vi "MagX Get Info From Server.vi"(6 "Save cache":bool, 7 "url":string="http://magx.lanl.gov/rest/now/", 8 "error in":errorcluster, 9 "Use cache":bool, 10 "Local cache  file":path=path "C:/Data/tmp/calendar.json", 11 "Station":string="Cell_3") -> (0 "error out":errorcluster, 2 "Online":bool, 3 "body":string)   [LabVIEW 2024]
uses:
  <vilib>/Utility/error.llb/Error Cluster From Error Code.vi
  <vilib>/ErrorRing/Error Ring.xnode
  <vilib>/httpClient/LabVIEWHTTPClient.lvlib
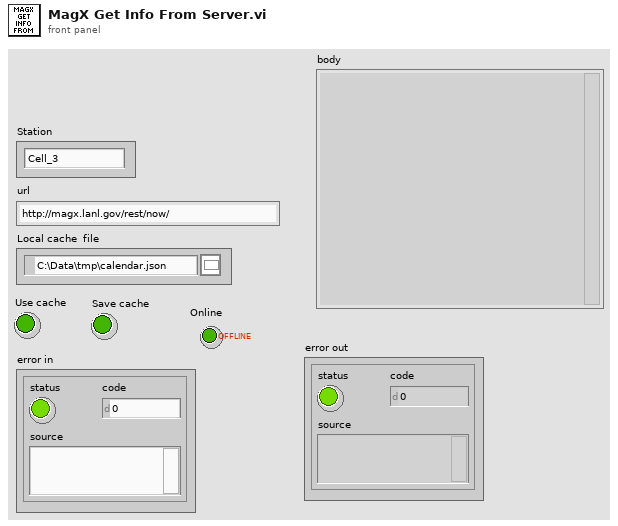
[diagram p1: front panel]
types:
  T1 = typedef "LabVIEWHTTPClient.lvlib/ClientHandle.ctl" = refnum<k1>
  T2 = enum16{"open", "replace", "create", "open or create", "replace or create", "replace or create with confirmation"}
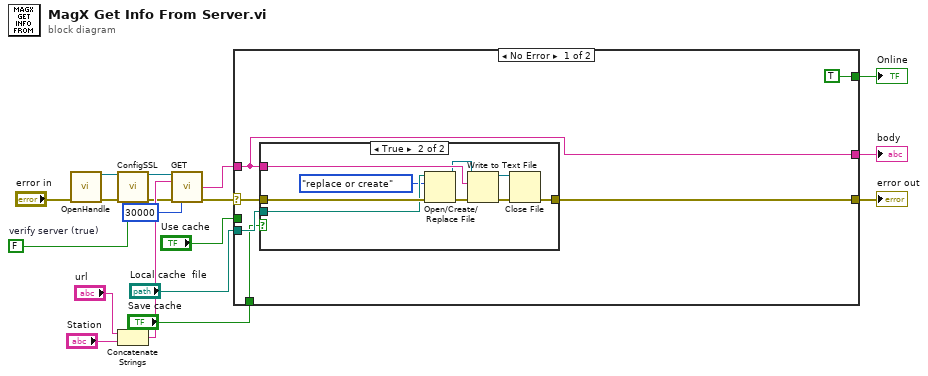
[diagram p0: block diagram]
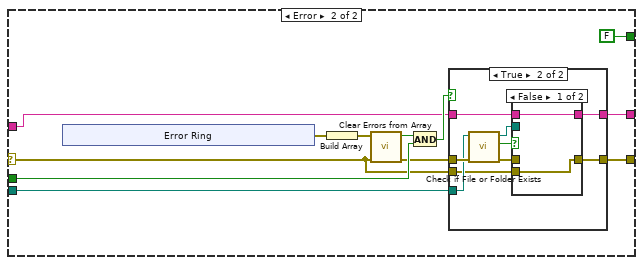
[diagram p3: hidden frame]
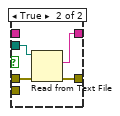
[diagram p5: hidden frame]
diagram:
  w10 = FALSE  # verify server (true)
  n1 = call <vilib>:"OpenHandle.vi"("error in (no error)"="error in") -> ("client handle out"=w14:T1, "error out"=w13:errorcluster)  [unwired: 13 in]
  n2 = call <vilib>:"ConfigSSL.vi"("client handle"=w14, "error in (no error)"=w13, "verify server (true)"=w10) -> ("client handle out"=w11:T1, "error out"=w12:errorcluster)  [unwired: 11 in]
  n3 = Concatenate Strings("url", "Station") -> (w17:string)
  n4 = call <vilib>:"GET.vi"("client handle"=w11, "url"=w17, "error in (no error)"=w12, "timeout (10000)"=30000) -> ("body"=w6:string, "error out"=w8:errorcluster)  [unwired: 8 in, 2 out]
  n5 = case shown="No Error" w8 {
    selector: w8 -> [w24 w38]
    tunnel: "Use cache" -> [_ w43]
    tunnel: "Local cache  file" -> [w23 w40]
    tunnel: w6 -> [w21 w36]
    tunnel: [w22 w39] -> w4
    tunnel: [w21 w37] -> w5
    tunnel: [TRUE FALSE] -> w3
    tunnel: "Save cache" -> [w19 _]
    frame No Error {
      n6 = case shown="True" w19 {
        tunnel: w24 -> [w25 w33]
        tunnel: w23 -> [_ w32]
        tunnel: w21 -> [_ w30]
        tunnel: [w25 w27] -> w22
        frame False {
        }
        frame True {
          n7 = Open/Create/Replace File(file path (use dialog)=w32, error in=w33, operation (0:open)=T2."replace or create") -> (refnum out=w26:refnum<file>, error out=w34:errorcluster)  [unwired: 3 in, 1 out]
          n8 = Write to Text File(file (use dialog)=w26, text=w30, error in=w34) -> (refnum out=w28:refnum<file>, error out=w29:errorcluster)  [unwired: 1 in, 1 out]
          n9 = Close File(refnum=w28, error in=w29) -> (error out=w27:errorcluster)  [unwired: 1 out]
        }
      }
    }
    frame Error {
      n10 = xnode "Error Ring"() -> ("error out"=w46:errorcluster)
      n11 = Build Array(w46) -> (w45:errorcluster[])
      n12 = call "Clear Errors from Array.vi"("Error In"=w38, "Errors to clear"=w45) -> ("Error Out"=w41:errorcluster, "specific error cleared?"=w44:bool)  [unwired: 8 in]
      n13 = And(x=w44, y=w43) -> (x .and. y?=w42:bool)
      n14 = case shown="True" w42 {
        tunnel: w41 -> [_ w57]
        tunnel: w40 -> [_ w56]
        tunnel: [w47 w53] -> w39
        tunnel: w38 -> [w47 w51]
        tunnel: [w48 w50] -> w37
        tunnel: w36 -> [w48 w49]
        frame False {
        }
        frame True {
          n15 = call <vilib>:"Check if File or Folder Exists.vi"("error in (no error)"=w57, "path"=w56) -> ("error out"=w54:errorcluster, "file or folder exists?"=w52:bool, "dup path"=w55:path)  [unwired: 7 in]
          n16 = case shown="False" w52 {
            tunnel: w55 -> [_ w63]
            tunnel: w54 -> [_ w62]
            tunnel: [w59 w61] -> w53
            tunnel: w51 -> [w59 _]
            tunnel: [w58 w60] -> w50
            tunnel: w49 -> [w58 _]
            frame False {
            }
            frame True {
              n17 = Read from Text File(file (use dialog)=w63, error in=w62) -> (text=w60:string, error out=w61:errorcluster)  [unwired: 2 in, 2 out]
            }
          }
        }
      }
    }
  }
  "body" <- w5
  "error out" <- w4
  "Online" <- w3
